vi "fgt get pressure Unit.vi"(8 "error in (no error)":errorcluster, 11 "pressureIndex":u32) -> (0 "error out":errorcluster, 3 "unit out":T1)   [LabVIEW 2020, in "fgt_SDK.lvlib"]
doc: "Get used unit on selected pressure device, default value is \"mbar\".\nEvery pressure read value and sent command use this unit."
uses:
  fgt_SDK.lvlib
  TypeDefs/fgt_PRESSURE_UNIT.ctl
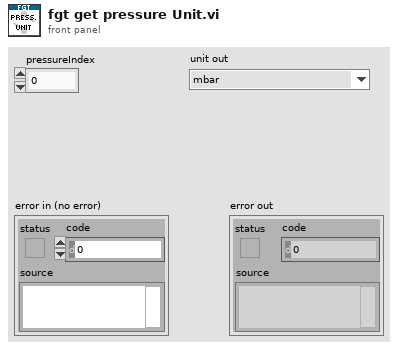
[diagram p1: front panel]
types:
  T1 = typedef "fgt_SDK.lvlib/fgt_PRESSURE_UNIT.ctl" = enum16{"mbar", "kPa", "PSI"}
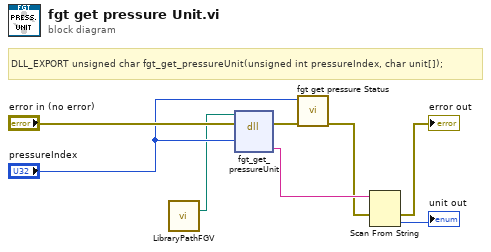
[diagram p0: block diagram]
diagram:
  # "DLL_EXPORT unsigned char fgt_get_pressureUnit(unsigned int pressureIndex, char unit[]);"
  n1 = call "LibraryPathFGV.vi"() -> ("Path Out"=w1:path)  [unwired: 14 in, 1 out]
  n2 = dll-call lib="C:/Workspace/fgt-SDK/LabVIEW/dlls/fgt_SDK_*.*" fn="fgt_get_pressureUnit"(path in=w1, error in="error in (no error)", "pressureIndex"="pressureIndex") -> (error out=w7:errorcluster, "unit"=w4:string)  [unwired: 4 in, 1 out]
  n3 = call "fgt get pressure Status.vi"("error in (no error)"=w7, "pressureIndex"="pressureIndex") -> ("error out"=w3:errorcluster)  [unwired: 9 in]
  n4 = Scan From String(input string=w4, error in=w3) -> (error out=→"error out":errorcluster, output 1=→"unit out":T1)  [unwired: 3 in, 2 out]
